vi "Autonomous Independent.vi"() -> ()   [LabVIEW 2012]
doc: "This VI is called when autonomous begins, and will automatically be terminated when autonomous ends. You can carry out timed or sensor driven robot movement independently without needing to return to the caller."
uses:
  <vilib>/Rock Robotics/WPI/Relay/WPI_RelayValue.ctl
  <vilib>/Rock Robotics/WPI/RobotDrive/WPI_RobotDriveGetSetRefNum.vi
  Robot Global Data.vi
panel:
  out "Shooter Speed":T1(ring)
  out "Stop Drive":bool
  out "DT Output":enum16{"Off", "Up", "Down"}(ring)=enum."Down"
  out "BAD Up":bool
  out "DAD Output":T2
  out "Shift Low":bool
  out "Feeder Happy":bool
  out "Auton Done":bool
  out "Shooter Happy":bool
  out "Shoot!":bool
  out "Loop Rate (Hz)":dbl
  out "Delay Switch":u32
  out "Seccond Switch":u32
  out "First Switch":u32
  # "Be sure to right-click and choose Data Operations>>Make Current Value default if you want to save the array values with the VI"
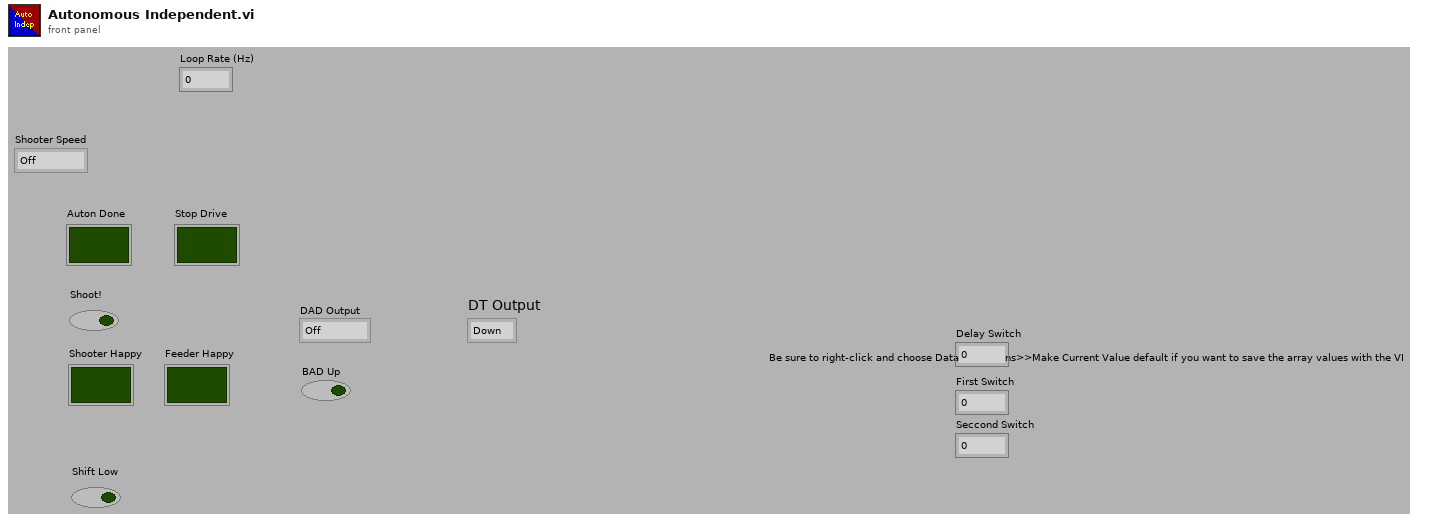
[diagram p1: front panel]
types:
  T1 = enum16{"Off", "Close Pyramid 3pt", "Far Pyramid 3pt", "Feeder Shot"}
  T2 = typedef "WPI_RelayValue.ctl" = enum16{"Off", "On", "Forward", "Reverse"}
  T3 = typedef "WPI_RobotDriveDevRef.ctl" = cluster{"DevStatus":errorcluster, "Motors[]":T4[], "Square Inputs":bool, "Max Output":dbl, "Isochronous":bool}
  T4 = typedef "WPI_MotorControlDeviceRef.ctl" = cluster{"DeviceStatus":errorcluster, "Type":enum16{"PWM", "CAN"}, "PWM":cluster{"Digital Module":T5, "PWM Channel":T6, "DeadBand":T7}, "CAN":cluster{"Device Number":u8, "Control Mode":T8, "Semaphore":T9, "Max Vout":dbl}, "Invert":bool, "TransformRef":T10, "InvTransformRef":T10}
  T5 = typedef "FPGA_TypedefDigitalModule.ctl" = enum16{"Digital Module 1", "Digital Module 2"}
  T6 = typedef "FPGA_DIOPWMChannel.ctl" = enum8{"PWM 1", "PWM 2", "PWM 3", "PWM 4", "PWM 5", "PWM 6", "PWM 7", "PWM 8", "PWM 9", "PWM 10", "Invalid"}
  T7 = typedef "WPI_PWMDeadband.ctl" = cluster{"Name":string, "maxPositivePwm":i32, "minPositivePwm":i32, "centerPwm":i32, "maxNegativePwm":i32, "minNegativePwm":i32, "angularRange":u16}
  T8 = typedef "WPI_CANJaguar_ControlMode.ctl" = enum8{"Percent VBus", "Current", "Speed", "Position", "Voltage"}
  T9 = typedef "Semaphore RefNum" = refnum<k1>
  T10 = typedef "WPI_PWMTransform_ConPane.ctl" = refnum<vi>
  T11 = typedef "WPI_GyroDevRef.ctl" = cluster{"DevStatus":errorcluster, "Analog Module":T12, "Analog Channel":T13, "Offset":dbl, "Gain (VoltsPerDegree/Second)":dbl}
  T12 = typedef "FPGA_TypedefAnalogModule.ctl" = enum16{"Analog Module 1", "Analog Module 2"}
  T13 = typedef "FPGA_AIChannel.ctl" = enum8{"AI 1", "AI 2", "AI 3", "AI 4", "AI 5", "AI 6", "AI 7", "AI 8", "Invalid"}
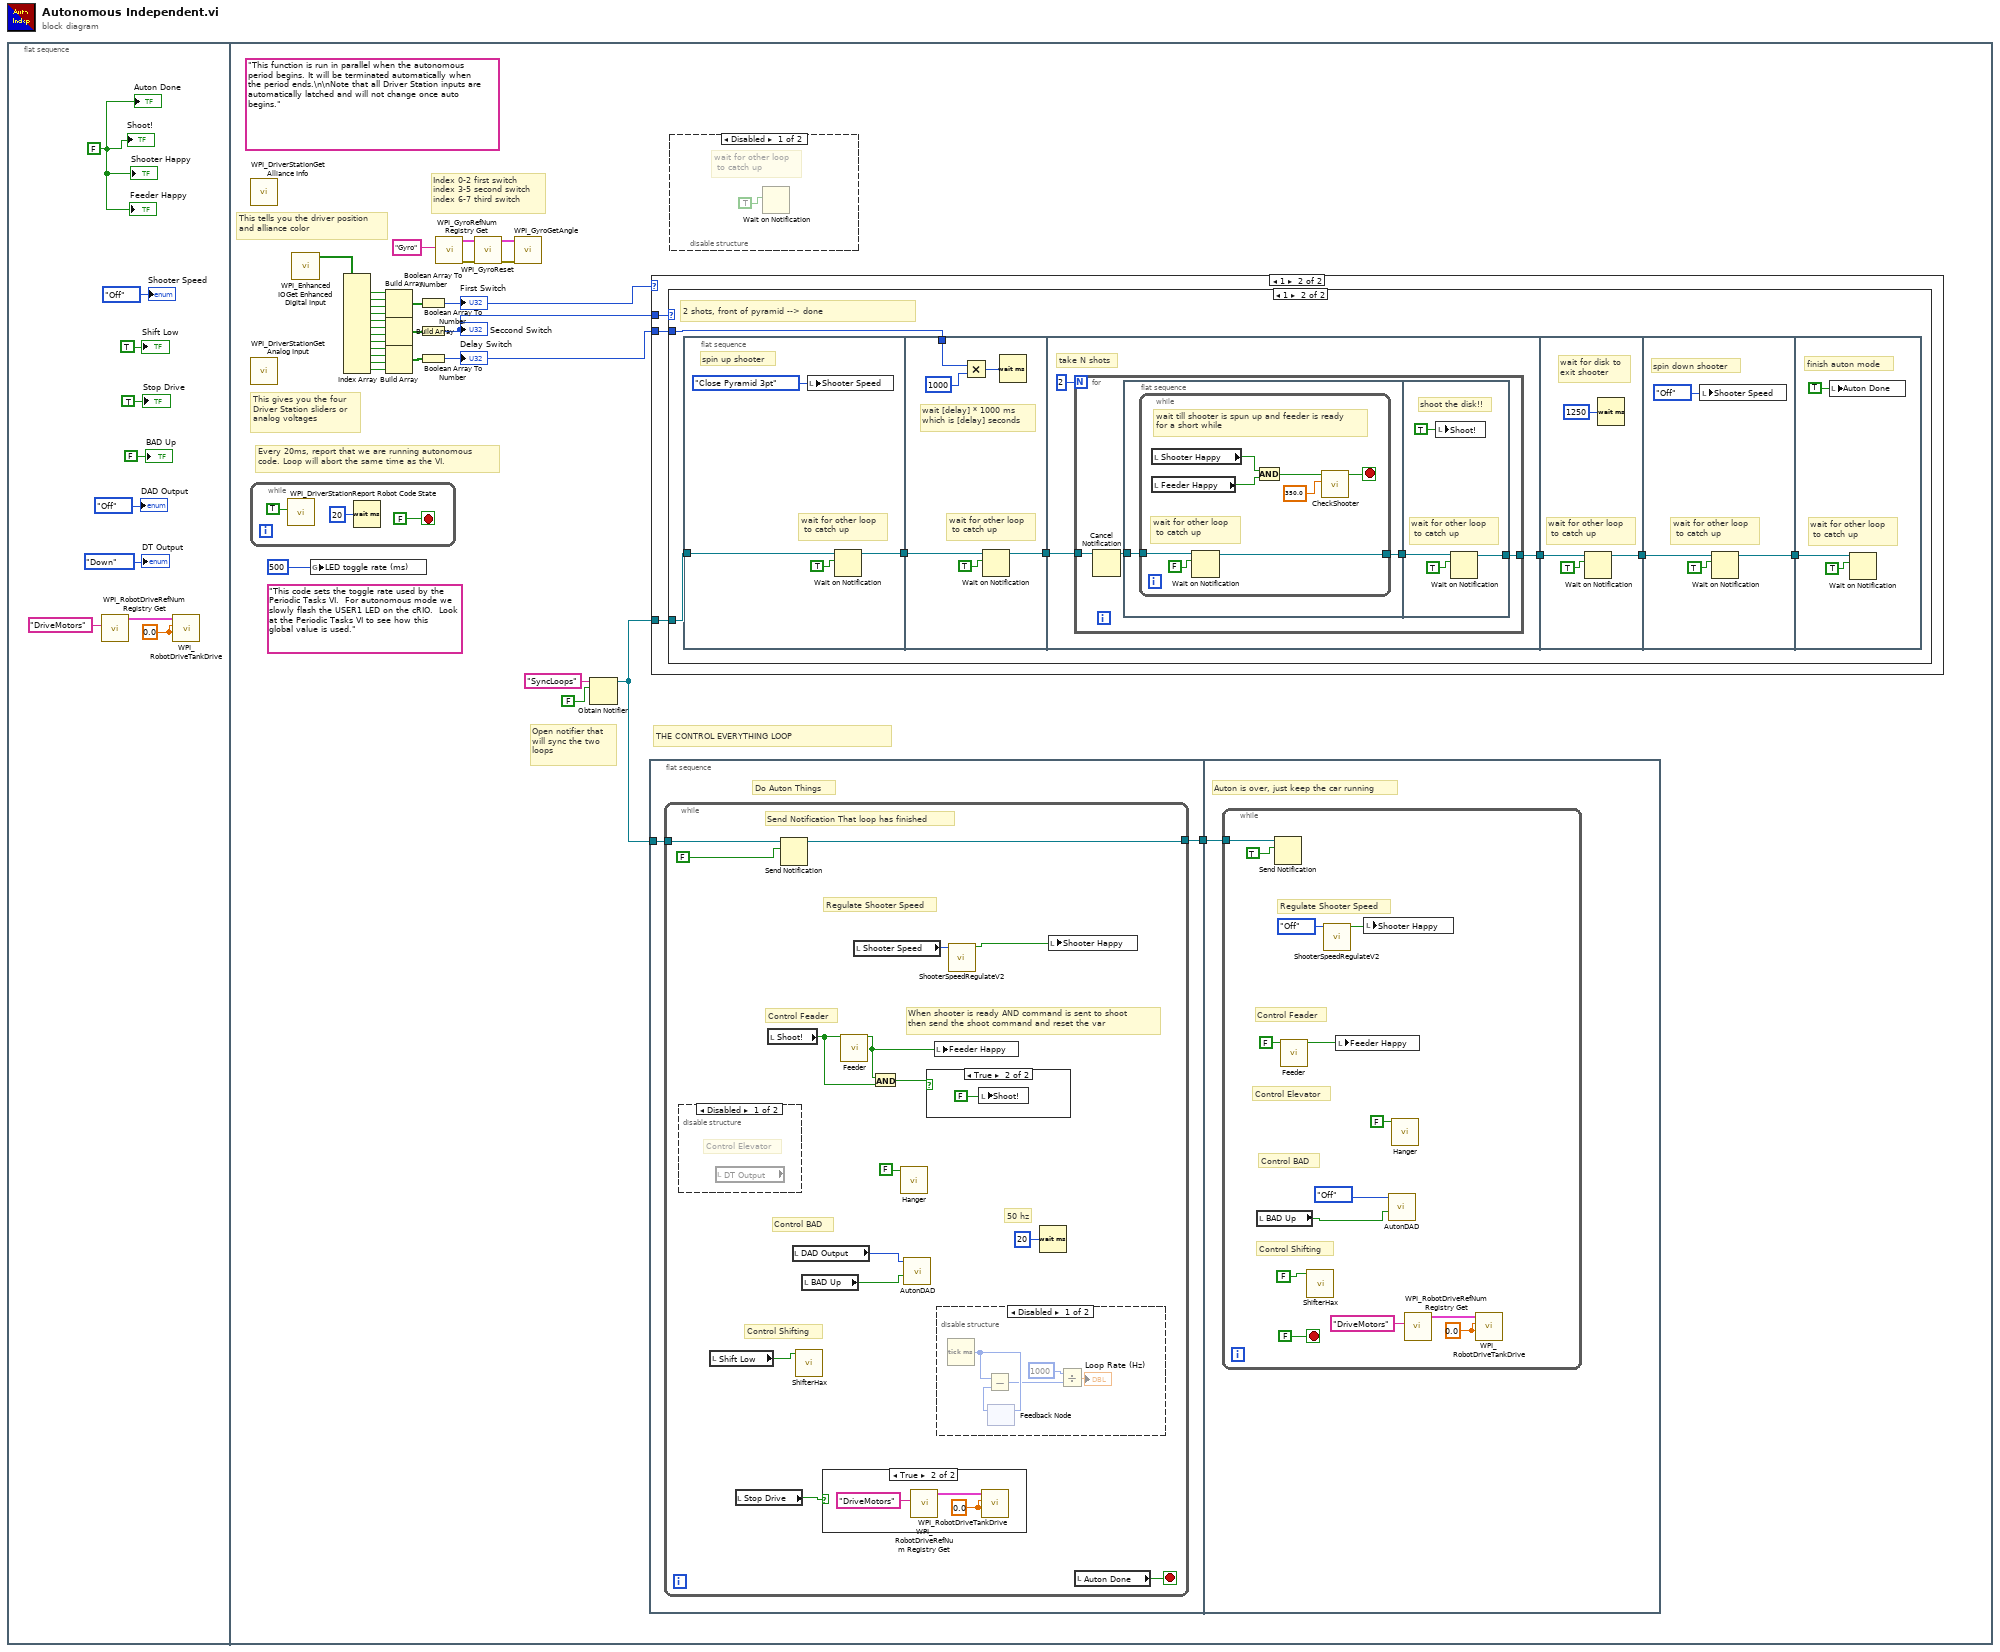
[diagram p0: block diagram]
diagram:
  n1 = flat-sequence {
    frame #0 {
      w3 = 0.0 ("Left axis value")
      w10 = FALSE
      n2 = call <vilib>:"WPI_RobotDriveRefNum Registry Get.vi"("refnum name"="DriveMotors") -> ("RobotDriveDevRef"=w5:T3)  [unwired: 1 in, 9 out]
      n3 = call <vilib>:"WPI_RobotDriveTankDrive.vi"("Right axis value"=w3, "Left axis value"=w3, "RobotDriveDevRef"=w5) -> ()  [unwired: 6 in, 3 out]
      "Feeder Happy" <- w10
      "Shift Low" <- TRUE ("Shift Low")
      "DAD Output" <- WPI_RelayValue."Off" ("DAD Output")
      "BAD Up" <- FALSE ("BAD Up")
      "Stop Drive" <- TRUE ("Stop Drive")
      "Shoot!" <- w10
      "Shooter Happy" <- w10
      "Auton Done" <- w10
      "DT Output" <- enum16{"Off", "Up", "Down"}."Down" ("DT Output")
      "Shooter Speed" <- T1."Off" ("Shooter Speed")
    }
    frame #1 {
      (unwired) "This code sets the toggle rate used by the Periodic Tasks VI.  For autonomous mode we slowly flash the USER1 LED on the cRIO.  Look at the Periodic Tasks VI to see how this global value is used."
      (unwired) "This function is run in parallel when the autonomous period begins. It will be terminated automatically when the period ends.\n\nNote that all Driver Station inputs are automatically latched and will not change once auto begins."
      # "THE CONTROL EVERYTHING LOOP"
      # "Index 0-2 first switch\nindex 3-5 second switch\nindex 6-7 third switch"
      # "Open notifier that\nwill sync the two\nloops"
      # "Every 20ms, report that we are running autonomous\ncode. Loop will abort the same time as the VI."
      # "This tells you the driver position\nand alliance color"
      # "This gives you the four\nDriver Station sliders or\nanalog voltages"
      n4 = call <vilib>:"WPI_DriverStationGet Alliance Info.vi"() -> ()  [unwired: 12 out]
      n5 = call <vilib>:"WPI_DriverStationGet Analog Input.vi"() -> ()  [unwired: 12 out]
      n6 = while {
        stop <- FALSE stop-if-true
        n7 = call <vilib>:"WPI_DriverStationReport Robot Code State.vi"("Autonomous"=TRUE) -> ()  [unwired: 10 in, 1 out]
        n8 = Wait (ms)(milliseconds to wait=u32 20) -> ()  [unwired: 1 out]
      }
      n9 = call <vilib>:"WPI_Enhanced IOGet Enhanced Digital Input.vi"() -> ("Digital Input [1-16]"=w15:bool[])  [unwired: 10 in, 1 out]
      n10 = global write "Robot Global Data.vi" "LED toggle rate (ms)"(u32 500 ("LED ms toggle rate")) -> ()
      n11 = Index Array(array=w15) -> (element #1=w35:bool, element #2=w34:bool, element #3=w33:bool, element #4=w21:bool, element #5=w32:bool, element #6=w31:bool, element #7=w23:bool, element #8=w22:bool, element #9=w20:bool, element #10=w19:bool, element #11=w18:bool, element #12=w17:bool)  [unwired: 12 in]
      n12 = Build Array(w35, w34, w33, w21) -> (w29:bool[])
      n13 = Build Array(w32, w31, w23, w22) -> (w30:bool[])
      n14 = Build Array(w20, w19, w18, w17) -> (w16:bool[])
      n15 = Boolean Array To Number(Boolean array=w29) -> (number=w14:u32)
      "First Switch" <- w14
      n16 = Boolean Array To Number(Boolean array=w30) -> (number=w13:u32)
      "Seccond Switch" <- w13
      n17 = Boolean Array To Number(Boolean array=w16) -> (number=w11:u32)
      "Delay Switch" <- w11
      n18 = call <vilib>:"WPI_GyroRefNum Registry Get.vi"("refnum name"="Gyro") -> ("error out"=w24:errorcluster, "GyroDevRef"=w25:T11)  [unwired: 9 in]
      n19 = call <vilib>:"WPI_GyroReset.vi"("error in (no error)"=w24, "GyroDevRef"=w25) -> ("error out"=w27:errorcluster, "GyroDevRef"=w26:T11)  [unwired: 8 in]
      n20 = call <vilib>:"WPI_GyroGetAngle.vi"("error in (no error)"=w27, "GyroDevRef"=w26) -> ()  [unwired: 6 in, 4 out]
      n21 = Obtain Notifier(name (unnamed)="SyncLoops", notification data type=FALSE) -> (notifier out=w12:refnum<notifier>)  [unwired: 2 in, 2 out]
      n22 = flat-sequence {
        tunnel: w12 -> [w43]
        tunnel: [w42] -> w39
        tunnel: w39 -> [w68]
        frame #0 {
          # "Do Auton Things"
          n23 = while {
            tunnel: w43 -> [w56]
            tunnel: [w52] -> w42
            stop <- w58 stop-if-true
            # "Regulate Shooter Speed"
            # "50 hz"
            # "Control BAD"
            # "Control Shifting"
            # "When shooter is ready AND command is sent to shoot\nthen send the shoot command and reset the var"
            # "Control Feader"
            # "Send Notification That loop has finished"
            n24 = disable-structure shown="Disabled" {
              frame Disabled {
                # "Control Elevator"
                n25 = local read "DT Output"() -> ()  [unwired: 1 out]
              }
              frame Enabled {
              }
            }
            n26 = local read "Shift Low"() -> (w46:bool)
            n27 = local read "Stop Drive"() -> (w50:bool)
            n28 = local read "Shoot!"() -> (w55:bool)
            n29 = Send Notification(notification=FALSE, notifier=w56) -> (notifier out=w52:refnum<notifier>)  [unwired: 1 in, 1 out]
            n30 = local read "DAD Output"() -> (w48:T2)
            n31 = call "ShifterHax.vi"("Shift low?"=w46) -> ()  [unwired: 11 in]
            n32 = local read "BAD Up"() -> (w49:bool)
            n33 = case shown="True" w50 {
              frame False {
              }
              frame True {
                w61 = 0.0 ("Left axis value")
                n34 = call <vilib>:"WPI_RobotDriveRefNum Registry Get.vi"("refnum name"="DriveMotors") -> ("RobotDriveDevRef"=w59:T3)  [unwired: 1 in, 9 out]
                n35 = call <vilib>:"WPI_RobotDriveTankDrive.vi"("Right axis value"=w61, "Left axis value"=w61, "RobotDriveDevRef"=w59) -> ()  [unwired: 6 in, 3 out]
              }
            }
            n36 = call "Feeder.vi"("SHOOT Button"=w55) -> ("Ready To Shoot?"=w53:bool)  [unwired: 10 in]
            n37 = local read "Shooter Speed"() -> (w45:T1)
            n38 = And(x=w53, y=w55) -> (x .and. y?=w54:bool)
            n39 = call "Hanger.vi"("Hanger Up"=FALSE) -> ()  [unwired: 10 in, 1 out]
            n40 = call "AutonDAD.vi"("BAD UP"=w49, "BAD Output"=w48) -> ()  [unwired: 10 in]
            n41 = case shown="True" w54 {
              frame False {
              }
              frame True {
                n42 = local write "Shoot!"(FALSE) -> ()
              }
            }
            n43 = local write "Feeder Happy"(w53) -> ()
            n44 = disable-structure shown="Disabled" {
              frame Disabled {
                n45 = Tick Count (ms)() -> (millisecond timer value=w66:u32)
                n46 = feedback #1() -> (w65:u32)  [unwired: 1 in]
                n47 = Subtract(x=w66, y=w65) -> (x-y=w63:u32)
                n48 = feedback-in #1(w66) -> ()
                n49 = Divide(x=1000, y=w63) -> (x/y=→"Loop Rate (Hz)":dbl)
              }
              frame Enabled {
              }
            }
            n50 = call "ShooterSpeedRegulateV2.vi"("Shooter Speed"=w45) -> ("ALL GOOD"=w47:bool)  [unwired: 13 in, 1 out]
            n51 = Wait (ms)(milliseconds to wait=u32 20) -> ()  [unwired: 1 out]
            n52 = local write "Shooter Happy"(w47) -> ()
            n53 = local read "Auton Done"() -> (w58:bool)
          }
        }
        frame #1 {
          # "Auton is over, just keep the car running"
          n54 = while {
            tunnel: w68 -> [w71]
            stop <- FALSE stop-if-true
            w77 = 0.0 ("Left axis value")
            # "Regulate Shooter Speed"
            # "Control BAD"
            # "Control Shifting"
            # "Control Elevator"
            # "Control Feader"
            n55 = local read "BAD Up"() -> (w74:bool)
            n56 = Send Notification(notification=TRUE, notifier=w71) -> ()  [unwired: 1 in, 2 out]
            n57 = call "Feeder.vi"("SHOOT Button"=FALSE) -> ("Ready To Shoot?"=w81:bool)  [unwired: 10 in]
            n58 = call "ShifterHax.vi"("Shift low?"=FALSE ("Shifting Button")) -> ()  [unwired: 11 in]
            n59 = call "ShooterSpeedRegulateV2.vi"("Shooter Speed"=T1."Off") -> ("ALL GOOD"=w76:bool)  [unwired: 13 in, 1 out]
            n60 = local write "Feeder Happy"(w81) -> ()
            n61 = local write "Shooter Happy"(w76) -> ()
            n62 = call "AutonDAD.vi"("BAD UP"=w74, "BAD Output"=WPI_RelayValue."Off") -> ()  [unwired: 10 in]
            n63 = call "Hanger.vi"("Hanger Up"=FALSE) -> ()  [unwired: 10 in, 1 out]
            n64 = call <vilib>:"WPI_RobotDriveRefNum Registry Get.vi"("refnum name"="DriveMotors") -> ("RobotDriveDevRef"=w79:T3)  [unwired: 1 in, 9 out]
            n65 = call <vilib>:"WPI_RobotDriveTankDrive.vi"("Right axis value"=w77, "Left axis value"=w77, "RobotDriveDevRef"=w79) -> ()  [unwired: 6 in, 3 out]
          }
        }
      }
      n66 = case shown="1" w14 {
        tunnel: w13 -> [_ w85]
        tunnel: w12 -> [_ w84]
        tunnel: w11 -> [_ w83]
        frame 0, Default {
          # "do nothing"
        }
        frame 1 {
          n67 = case shown="1" w85 {
            tunnel: w84 -> [_ w89]
            tunnel: w83 -> [_ w92]
            frame 0, Default {
              # "do nothing"
            }
            frame 1 {
              # "2 shots, front of pyramid --> done"
              n68 = flat-sequence {
                tunnel: [w95] -> w91
                tunnel: w89 -> [w94]
                tunnel: w92 -> [w100]
                tunnel: w91 -> [w98]
                tunnel: [w97] -> w90
                tunnel: w90 -> [w104]
                tunnel: [w103] -> w86
                tunnel: [w125] -> w87
                tunnel: w86 -> [w124]
                tunnel: [w130] -> w88
                tunnel: w87 -> [w129]
                tunnel: w88 -> [w132]
                frame #0 {
                  # "wait for other loop\n to catch up"
                  # "spin up shooter"
                  n69 = local write "Shooter Speed"(T1."Close Pyramid 3pt" ("Shooter Speed")) -> ()
                  n70 = Wait on Notification(notifier=w94, ignore previous (F)=TRUE) -> (notifier out=w95:refnum<notifier>)  [unwired: 2 in, 3 out]
                }
                frame #1 {
                  # "wait for other loop\n to catch up"
                  # "wait [delay] * 1000 ms\nwhich is [delay] seconds"
                  n71 = Multiply(x=w100, y=1000) -> (x*y=w102:u32)
                  n72 = Wait on Notification(notifier=w98, ignore previous (F)=TRUE) -> (notifier out=w97:refnum<notifier>)  [unwired: 2 in, 3 out]
                  n73 = Wait (ms)(milliseconds to wait=w102) -> ()  [unwired: 1 out]
                }
                frame #2 {
                  # "take N shots"
                  n74 = for {
                    N: 2 -> [_]
                    tunnel: w104 -> [w108]
                    tunnel: [w106] -> w103
                    n75 = Cancel Notification(0:w108) -> (8:w109:refnum<notifier>)  [unwired: 1 in, 2 out]
                    n76 = flat-sequence {
                      tunnel: w109 -> [w111]
                      tunnel: [w110] -> w107
                      tunnel: w107 -> [w121]
                      tunnel: [w120] -> w106
                      frame #0 {
                        n77 = while {
                          tunnel: w111 -> [w113]
                          tunnel: [w112] -> w110
                          stop <- w115 stop-if-true
                          # "wait for other loop\n to catch up"
                          # "wait till shooter is spun up and feeder is ready\nfor a short while"
                          n78 = local read "Shooter Happy"() -> (w118:bool)
                          n79 = local read "Feeder Happy"() -> (w117:bool)
                          n80 = Wait on Notification(notifier=w113, ignore previous (F)=FALSE) -> (notifier out=w112:refnum<notifier>)  [unwired: 2 in, 3 out]
                          n81 = And(x=w118, y=w117) -> (x .and. y?=w116:bool)
                          n82 = call "CheckShooter.vi"("Time for happy (ms)"=350.0, "Shooter Good?"=w116) -> ("Good to shoot"=w115:bool)  [unwired: 9 in]
                        }
                      }
                      frame #1 {
                        # "wait for other loop\n to catch up"
                        # "shoot the disk!!"
                        n83 = local write "Shoot!"(TRUE ("Shoot!")) -> ()
                        n84 = Wait on Notification(notifier=w121, ignore previous (F)=TRUE) -> (notifier out=w120:refnum<notifier>)  [unwired: 2 in, 3 out]
                      }
                    }
                  }
                }
                frame #3 {
                  # "wait for other loop\n to catch up"
                  # "wait for disk to\nexit shooter"
                  n85 = Wait on Notification(notifier=w124, ignore previous (F)=TRUE) -> (notifier out=w125:refnum<notifier>)  [unwired: 2 in, 3 out]
                  n86 = Wait (ms)(milliseconds to wait=u32 1250) -> ()  [unwired: 1 out]
                }
                frame #4 {
                  # "wait for other loop\n to catch up"
                  # "spin down shooter"
                  n87 = local write "Shooter Speed"(T1."Off" ("Shooter Speed")) -> ()
                  n88 = Wait on Notification(notifier=w129, ignore previous (F)=TRUE) -> (notifier out=w130:refnum<notifier>)  [unwired: 2 in, 3 out]
                }
                frame #5 {
                  # "wait for other loop\n to catch up"
                  # "finish auton mode"
                  n89 = local write "Auton Done"(TRUE ("Auton Done")) -> ()
                  n90 = Wait on Notification(notifier=w132, ignore previous (F)=TRUE) -> ()  [unwired: 2 in, 4 out]
                }
              }
            }
          }
        }
      }
      n91 = disable-structure shown="Disabled" {
        frame Disabled {
          # "wait for other loop\n to catch up"
          n92 = Wait on Notification(ignore previous (F)=TRUE) -> (notifier=w41:refnum<notifier>)  [unwired: 2 in, 4 out]
        }
        frame Enabled {
        }
      }
    }
  }
